vi "DeltaT_2_Power.vi"(8 "Longueur d'onde":dbl, 10 "Delta T":dbl) -> (2 "Power":dbl)   [LabVIEW 2018]
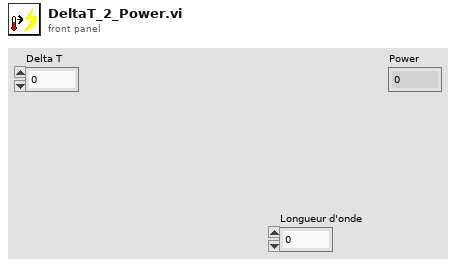
[diagram p1: front panel]
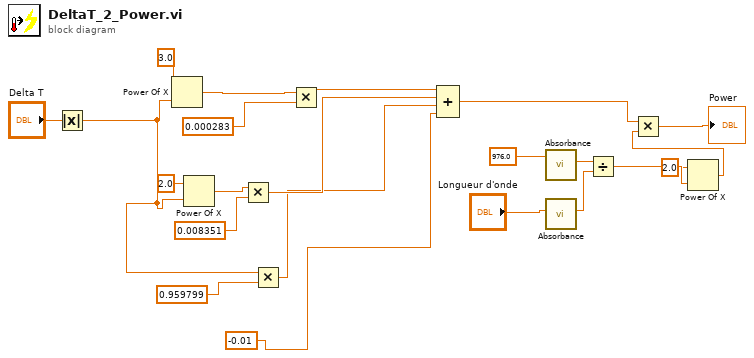
[diagram p0: block diagram]
diagram:
  n1 = Absolute Value(x="Delta T") -> (abs(x)=w15:dbl)
  n2 = Power Of X(1:w15, 2:3.0 ("y")) -> (0:w19:dbl)
  n3 = Power Of X(1:w15, 2:2.0 ("y")) -> (0:w20:dbl)
  n4 = Multiply(x=w20, y=0.008351 ("x")) -> (x*y=w17:dbl)
  n5 = Multiply(x=w15, y=0.959799 ("x")) -> (x*y=w16:dbl)
  n6 = Multiply(x=w19, y=0.000283 ("x")) -> (x*y=w18:dbl)
  n7 = Compound Arithmetic op=ADD(w18, w17, w16, -0.01 ("x")) -> (w9:dbl)
  n8 = call "Absorbance.vi"("Longueur d'onde"=976.0) -> ("absorbance"=w11:dbl)  [unwired: 10 in]
  n9 = call "Absorbance.vi"("Longueur d'onde"="Longueur d'onde") -> ("absorbance"=w10:dbl)  [unwired: 10 in]
  n10 = Divide(x=w11, y=w10) -> (x/y=w3:dbl)
  n11 = Power Of X(1:w3, 2:2.0 ("y")) -> (0:w1:dbl)
  n12 = Multiply(x=w9, y=w1) -> (x*y=→"Power":dbl)
